vi "Attenuator Write to INI File.vi"(4 "Step Number":i32=1, 7 "Display":T1={"Lock Control"=FALSE, "Retain Settings"=TRUE, "Formatted Data"=FALSE, "Plot Orientation"=enum."Single", "Plot Controls"=[{"Trace Orientation"=enum."Overlay", "Frequency"={"Change Frequency"=FALSE, "Start"=500.0, "Stop"=1500.0, "Units"=enum."MHz"}, "Markers"=[], "Traces"=[]}, {"Trace Orientation"=enum."Overlay", "Frequency"={"Change Frequency"=FALSE, "Start"=500.0, "Stop"=1500.0, "Units"=enum."MHz"}, "Markers"=[], "Traces"=[]}, {"Trace Orientation"=enum."Overlay", "Frequency"={"Change Frequency"=FALSE, "Start"=500.0, "Stop"=1500.0, "Units"=enum."MHz"}, "Markers"=[], "Traces"=[]}, {"Trace Orientation"=enum."Overlay", "Frequency"={"Change Frequency"=FALSE, "Start"=500.0, "Stop"=1500.0, "Units"=enum."MHz"}, "Markers"=[], "Traces"=[]}]} {"Plot Controls"."Traces"."Reference" format="%#.2g"; "Plot Controls"."Traces"."Display Data" items=["Data", "Memory", "Data/Memory"]; "Plot Controls"."Traces"."Format" items=["Log Mag", "Phase", "Expanded Phase", "Delay", "Smith", "Polar", "Lin Mag", "SWR", "Loss", "Real", "Imaginary"]; "Plot Controls"."Traces"."Scale" min=0.001 step=1.0 format="%#.2g"; "Plot Controls"."Traces"."Position" min=0.0 max=10.0; "Plot Controls"."Frequency"."Stop" format="%.3g"; "Plot Controls"."Frequency"."Start" format="%.3g"}, 8 "error in (no error)":errorcluster, 9 "Requested Stimulus":T9={"ATT Stimulus"={"Normalize"=TRUE, "Value (dB)"=0.0}, "VNA Stimulus"={"Use Instrument Settings"=FALSE, "Blank Frequencies"=FALSE, "Sweep Type"=enum."Linear", "Sweep"={"Fstart"=500.0, "Fstop"=1500.0, "Units"=enum."MHz", "Points"=201}, "Power (dBm)"=999.0, "IFBW (Hz)"=-1.0, "Sweep Time (s)"=-1.0, "Calibration"={"State"=FALSE, "String"=""}}} {"VNA Stimulus"."Sweep Time (s)" format="%.3g"}, 10 "Parameters to Measure":T13[](array[typedef]) {"Channel" min=1 max=99 step=1; "Parameter"."Stimulus Port" min=1 step=1; "Parameter"."Response Port" min=1 step=1}, 11 "Data to Write":enum16{"Calibration", "Display"}(ring)) -> (0 "error out":errorcluster)   [LabVIEW 2011]
uses:
  TypeDefs/Attenuator Parameter to Measure.ctl
  S Parameter/TypeDefs/SP Parameter.ctl
  TypeDefs/Attenuator VNA Calibration State.ctl
  S Parameter/TypeDefs/SP Measurement Format.ctl
  TypeDefs/Attenuator Stimulus Parameters.ctl
  TypeDefs/Attenuator ATT Stimulus.ctl
  TypeDefs/Attenuator VNA Stimulus.ctl
  S Parameter/TypeDefs/SP Frequency Units.ctl
  S Parameter/TypeDefs/SP Display Parameters.ctl
  S Parameter/TypeDefs/SP Display Plot Controls Cluster.ctl
  S Parameter/TypeDefs/SP Marker Cluster.ctl
  S Parameter/TypeDefs/SP Marker Type.ctl
  S Parameter/TypeDefs/SP Display Trace Controls.ctl
  S Parameter/TypeDefs/SP Display Format.ctl
  S Parameter/TypeDefs/SP Display Data.ctl
  <vilib>/Utility/config.llb/Write Key (String).vi
  <vilib>/Utility/config.llb/NI_LVConfig.lvlib
panel:
  # "Div"
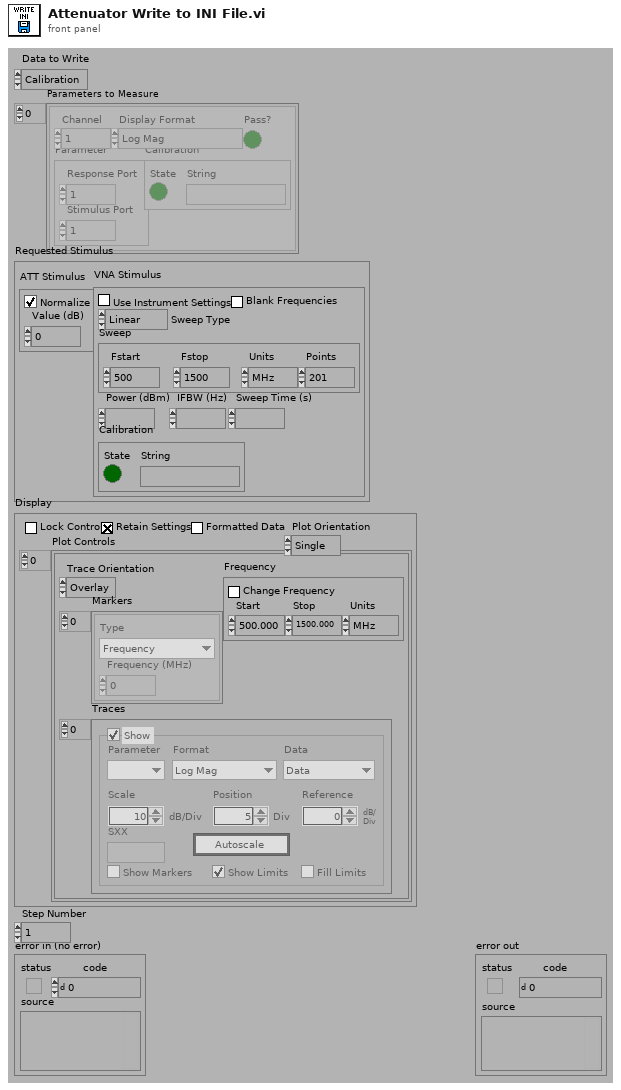
[diagram p1: front panel]
types:
  T1 = typedef "SP Display Parameters.ctl" = cluster{"Lock Control":bool, "Retain Settings":bool, "Formatted Data":bool, "Plot Orientation":enum32{"Single", "Dual", "Quad"}, "Plot Controls":T2[]}
  T2 = typedef "SP Display Plot Controls Cluster.ctl" = cluster{"Trace Orientation":enum32{"Overlay", "Split"}, "Frequency":cluster{"Change Frequency":bool, "Start":dbl, "Stop":dbl, "Units":T3}, "Markers":T4[], "Traces":T6[]}
  T3 = typedef "SP Frequency Units.ctl" = enum16{"Hz", "kHz", "MHz", "GHz", "Points"}
  T4 = typedef "SP Marker Cluster.ctl" = cluster{"Type":T5, "Frequency (MHz)":dbl}
  T5 = typedef "SP Marker Type.ctl" = enum16{"Frequency", "Trace Maximum", "Trace Minimum", "Limit Maximum", "Limit Minimum"}
  T6 = typedef "SP Display Trace Controls.ctl" = cluster{"Trace On":bool, "Measure":i32, "Format":T7, "Autoscale":bool, "Reference":dbl, "\nRefUnit":string, "Position":dbl, "Scale":dbl, "ScaleUnit":string, "LimitOn":bool, "LimitFill":bool, "Display Data":T8, "Show Markers":bool, "SXX":string}
  T7 = typedef "SP Display Format.ctl" = i32
  T8 = typedef "SP Display Data.ctl" = u16
  T9 = typedef "Attenuator Stimulus Parameters.ctl" = cluster{"ATT Stimulus":T10, "VNA Stimulus":T11}
  T10 = typedef "Attenuator ATT Stimulus.ctl" = cluster{"Normalize":bool, "Value (dB)":dbl}
  T11 = typedef "Attenuator VNA Stimulus.ctl" = cluster{"Use Instrument Settings":bool, "Blank Frequencies":bool, "Sweep Type":enum32{"Linear", "Logarithmic", "List", "Power", "CW"}, "Sweep":cluster{"Fstart":dbl, "Fstop":dbl, "Units":T3, "Points":i32}, "Power (dBm)":dbl, "IFBW (Hz)":dbl, "Sweep Time (s)":dbl, "Calibration":T12}
  T12 = typedef "Attenuator VNA Calibration State.ctl" = cluster{"State":bool, "String":string}
  T13 = typedef "Attenuator Parameter to Measure.ctl" = cluster{"Channel":i8, "Parameter":T14, "Calibration":T12, "Display Format":T15, "Pass?":bool}
  T14 = typedef "SP Parameter.ctl" = cluster{"Stimulus Port":i8, "Response Port":i8}
  T15 = typedef "SP Measurement Format.ctl" = enum32{"Log Mag", "Phase", "Delay", "Smith (R+jX)", "Polar (Re/Im)", "Linear Mag", "SWR", "Real", "Imaginary", "Smith (Lin/Phase)", "Smith (Log/Phase)", "Smith (Real/Imag)", "Smith (G+jB)", "Polar (Lin/Phase)", "Polar (Log/Phase)", "Expanded Phase", "Positive Phase", "Inverted Smith", "Unwrapped Phase", "Power Out", "Power In", "Linear Mag/Phase", "Log Mag/Phase", "Real/Imaginary"}
  T16 = typedef "NI_LVConfig.lvlib/Config Data RefNum.ctl" = refnum<k1>
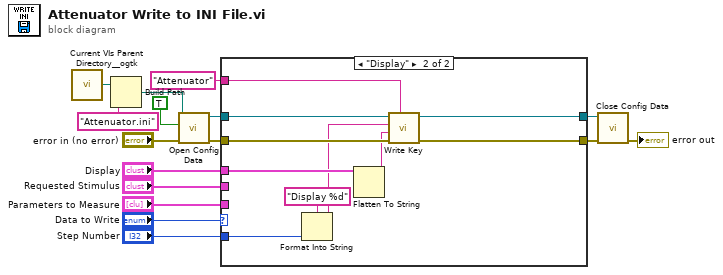
[diagram p0: block diagram]
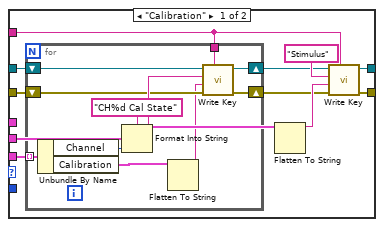
[diagram p2: hidden frame]
diagram:
  n1 = call "Current VIs Parent Directory__ogtk.vi"() -> ("Parent Directory (+ Relative)"=w1:path)  [unwired: 5 in]
  n2 = Build Path(base path=w1, name or relative path="Attenuator.ini") -> (appended path=w3:path)
  n3 = call <vilib>:"Open Config Data.vi"("error in (no error)"="error in (no error)", "create file if necessary (T)"=TRUE ("create file if necessary? (T)"), "configuration file path"=w3) -> ("error out"=w10:errorcluster, "refnum"=w9:T16)  [unwired: 6 in, 1 out]
  n4 = case shown="\"Display\"" "Data to Write" {
    tunnel: [w26 w43] -> w14
    tunnel: [w25 w44] -> w13
    tunnel: w10 -> [w22 w48]
    tunnel: w9 -> [w21 w47]
    tunnel: "Parameters to Measure" -> [w18 _]
    tunnel: "Requested Stimulus" -> [w23 _]
    tunnel: "Attenuator" ("section") -> [w17 w46]
    tunnel: "Display" -> [_ w45]
    tunnel: "Step Number" -> [_ w41]
    frame "Calibration" {
      n5 = for {
        tunnel: w18 -> [w37] mode=indexing
        shift-right: [w34] -> w19
        shift-left: w22 -> [w35]
        shift-right: [w33] -> w20
        shift-left: w21 -> [w32]
        tunnel: w17 -> [w31]
        n6 = Unbundle By Name(w37) -> ("Channel"=w28:i8, "Calibration"=w30:T12)
        n7 = Format Into String(format string="CH%d Cal State", w28) -> (resulting string=w36:string)  [unwired: 2 in, 1 out]
        n8 = Flatten To String(anything=w30) -> (data string=w29:string)  [unwired: 1 in, 4 out]
        n9 = call-poly <vilib>:"Write Key.vi"("section"=w31, "error in (no error)"=w35, "value"=w29, "key"=w36, "refnum"=w32) -> ("error out"=w34:errorcluster, "refnum out"=w33:T16)  [unwired: 1 in, 4 out]
      }
      n10 = Flatten To String(anything=w23) -> (data string=w27:string)  [unwired: 1 in, 4 out]
      n11 = call-poly <vilib>:"Write Key.vi"("section"=w17, "error in (no error)"=w19, "value"=w27, "key"="Stimulus", "refnum"=w20) -> ("error out"=w25:errorcluster, "refnum out"=w26:T16)  [unwired: 1 in, 4 out]
    }
    frame "Display" {
      n12 = Format Into String(format string="Display %d" ("section"), w41) -> (resulting string=w39:string)  [unwired: 2 in, 1 out]
      n13 = Flatten To String(anything=w45) -> (data string=w42:string)  [unwired: 1 in, 4 out]
      n14 = call-poly <vilib>:"Write Key.vi"("section"=w46, "error in (no error)"=w48, "value"=w42, "key"=w39, "refnum"=w47) -> ("error out"=w44:errorcluster, "refnum out"=w43:T16)  [unwired: 1 in, 4 out]
    }
  }
  n15 = call <vilib>:"Close Config Data.vi"("error in (no error)"=w13, "refnum"=w14) -> ("error out"=→"error out":errorcluster)  [unwired: 1 in, 8 out]
